vi "Initialize Parameter File.vi"(6 "File type":enum16{"INI"}(ring), 7 "Section":string, 8 "error in (no error)":errorcluster, 9 "create file if necessary (T)":bool=TRUE, 10 "configuration file path (blank opens dialog)":path, 11 "CD Parameter Manager in":refnum<class "CD Parameter Manager.lvclass">) -> (0 "error out":errorcluster, 3 "CD Parameter Manager out":refnum<class "CD Parameter Manager.lvclass">)   [LabVIEW 2016, in "CD Parameter Manager API.lvlib" / "CD Parameter Manager.lvclass"]
uses:
  CD Parameter Manager.lvclass
  Parameter INI File/Parameter INI File.lvclass
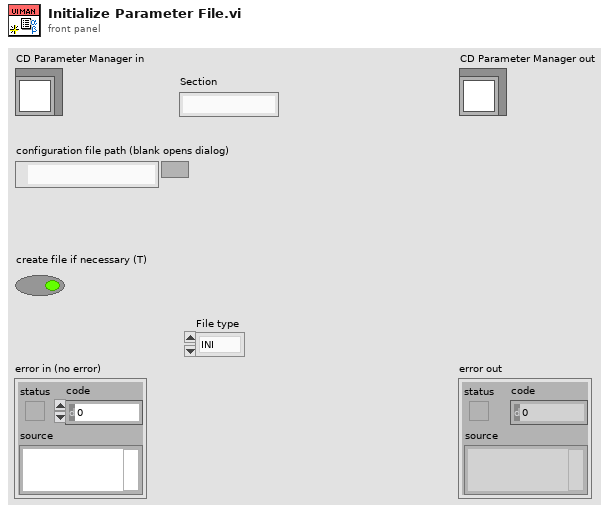
[diagram p1: front panel]
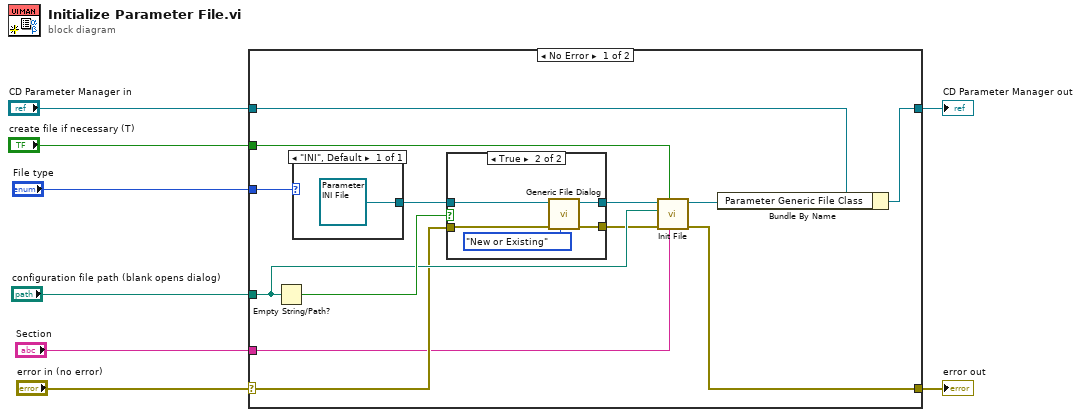
[diagram p0: block diagram]
diagram:
  n1 = case shown="No Error" "error in (no error)" {
    selector: "error in (no error)" -> [w16 w31]
    tunnel: [w12 w31] -> w7
    tunnel: [w9 w30] -> w5
    tunnel: "CD Parameter Manager in" -> [w15 w30]
    tunnel: "File type" -> [w21 _]
    tunnel: "configuration file path (blank opens dialog)" -> [w17 _]
    tunnel: "create file if necessary (T)" -> [w11 _]
    tunnel: "Section" -> [w10 _]
    frame No Error {
      n2 = Empty String/Path?(string/path=w17) -> (empty?=w20:bool)
      n3 = case shown="\"INI\", Default" w21 {
        tunnel: [refnum<class "Parameter INI File.lvclass"> refnum ("CD Parameter Manager API.lvlib:Parameter INI File.lvclass")] -> w19
        frame "INI", Default {
        }
      }
      n4 = case shown="True" w20 {
        tunnel: w19 -> [w23 w28]
        tunnel: [w23 w27] -> w18
        tunnel: w16 -> [w22 w26]
        tunnel: [w22 w25] -> w13
        frame False {
        }
        frame True {
          n5 = call-dynamic "Generic File Dialog.vi"("Selection mode"=enum16{"New", "Existing", "New or Existing"}."New or Existing", "error in (no error)"=w26, "Parameter INI File in"=w28) -> ("error out"=w25:errorcluster, "Parameter INI File out"=w27:refnum<class "Parameter INI File.lvclass">)  [unwired: 7 in]
        }
      }
      n6 = call-dynamic "Init File.vi"("Section"=w10, "create file if necessary (T)"=w11, "error in (no error)"=w13, "configuration file path"=w17, "Parameter INI File in"=w18) -> ("error out"=w12:errorcluster, "Parameter INI File out"=w14:refnum<class "Parameter INI File.lvclass">)  [unwired: 5 in]
      n7 = Bundle By Name(cluster=w15, "Parameter Generic File Class"=w14) -> (w9:refnum<class "CD Parameter Manager.lvclass">)
    }
    frame Error {
    }
  }
  "error out" <- w7
  "CD Parameter Manager out" <- w5
